vi "prepare_inserts_for_save_results.vi"(6 "operation_ID":string, 7 "SQL_connection_reference":T1, 8 "error_in":errorcluster, 9 "station":T2, 10 "results_from_PLC":T3, 11 "archivisation_info":string[][](array[string])) -> (0 "error_out":errorcluster, 3 "INSERT_statements":string[](array[string]), 5 "All PART_NUMBERS exist?":bool)   [LabVIEW 2020]
uses:
  ST_results_info.ctl
  station.ctl
  <vilib>/addons/database/Connection.llb/Conn ObjectReference.ctl
  FGV/SQL_batch_ID_buffer/FGV_SQL_batch_ID_buffer.ctl
  _misc/AULocalize/SubVIs/Get Localized Phrase Compact Interface 0D.vi
  <vilib>/addons/database/NI_Database_API.lvlib
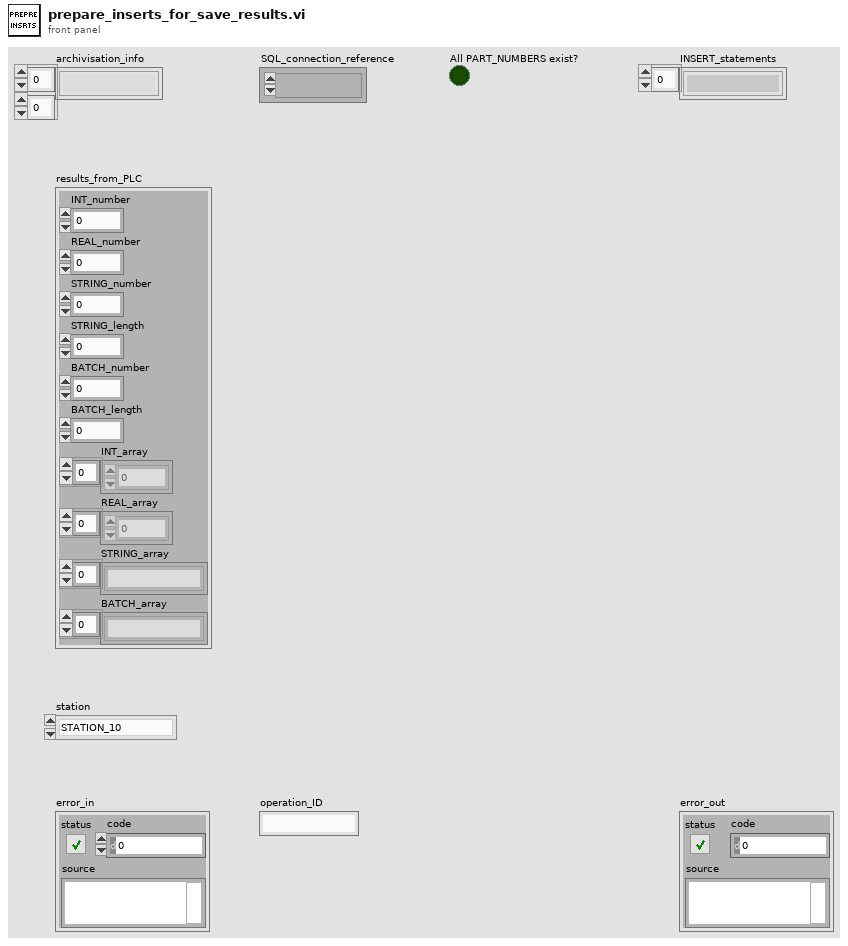
[diagram p1: front panel]
types:
  T1 = typedef "NI_Database_API.lvlib/Conn ObjectReference.ctl" = refnum<k1>
  T2 = typedef "station.ctl" = enum16{"STATION_10", "STATION_20", "STATION_30", "STATION_40", "STATION_50", "STATION_60", "STATION_70", "STATION_80", "STATION_90", "STATION_100", "STATION_110", "STATION_120", "STATION_165", "MAIN"}
  T3 = typedef "ST_results_info.ctl" = cluster{"INT_number":i32, "REAL_number":i32, "STRING_number":i32, "STRING_length":i32, "BATCH_number":i32, "BATCH_length":i32, "INT_array":i16[], "REAL_array":sgl[], "STRING_array":string[], "BATCH_array":string[]}
  T4 = typedef "FGV_SQL_batch_ID_buffer.ctl" = enum16{"initialize", "get_ID_for_number"}
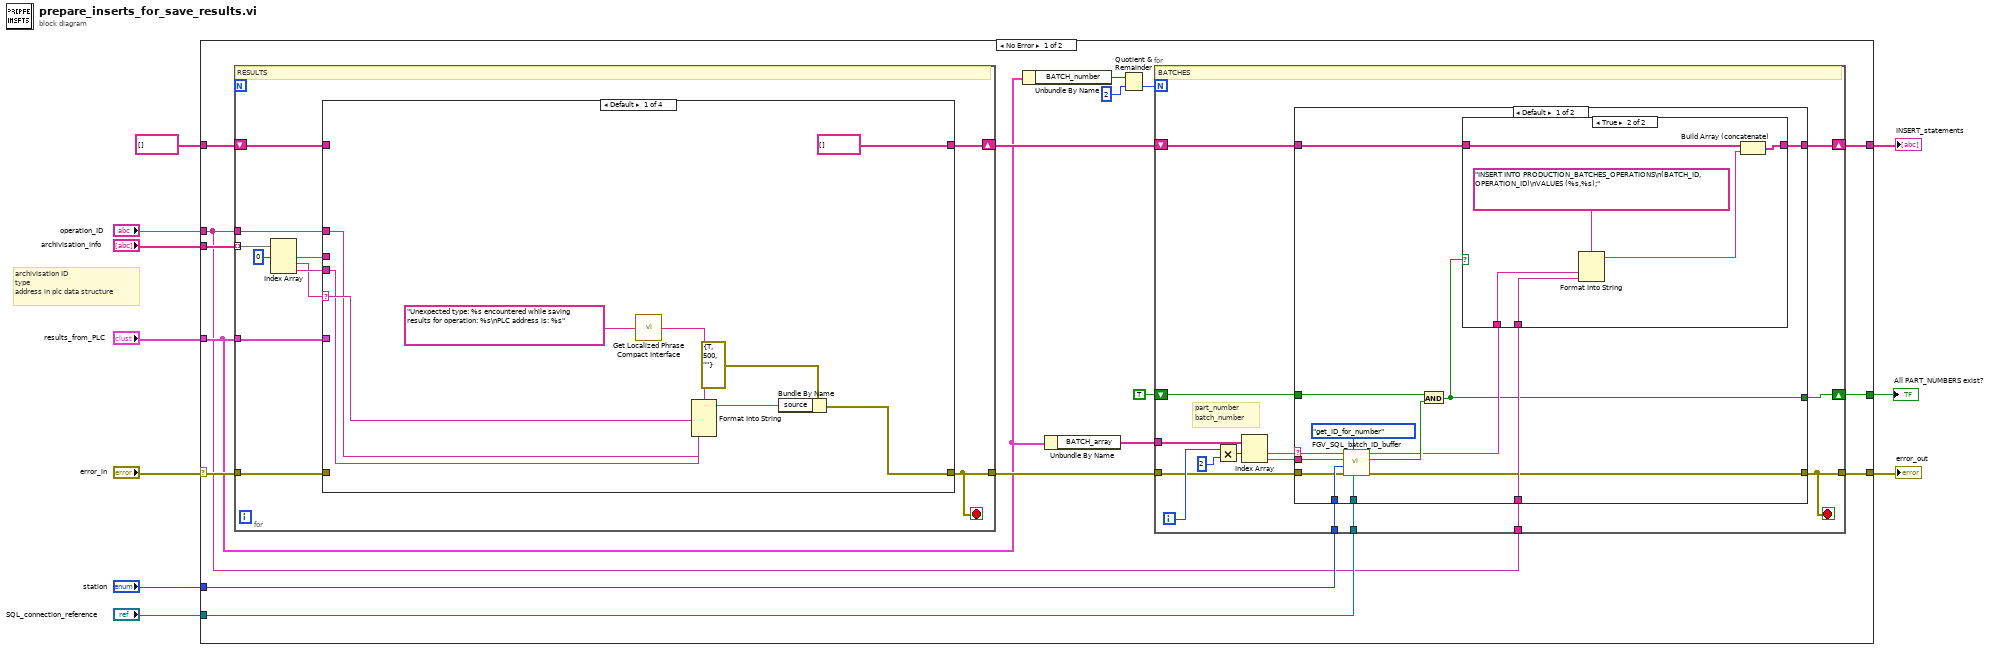
[diagram p0: block diagram]
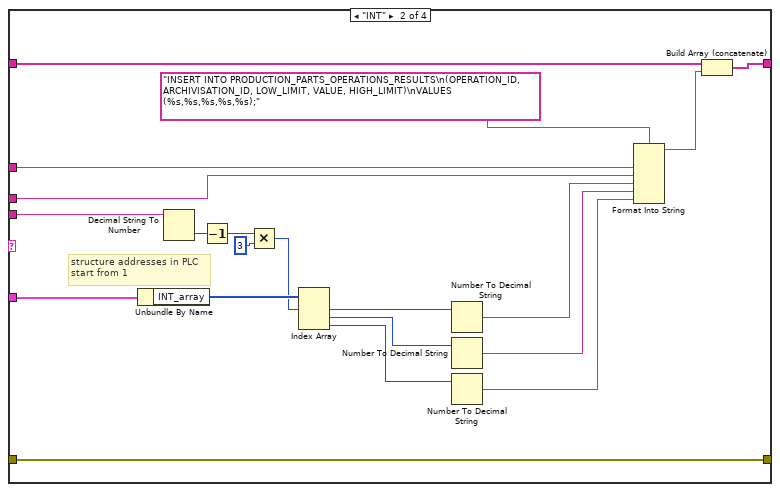
[diagram p4: hidden frame]
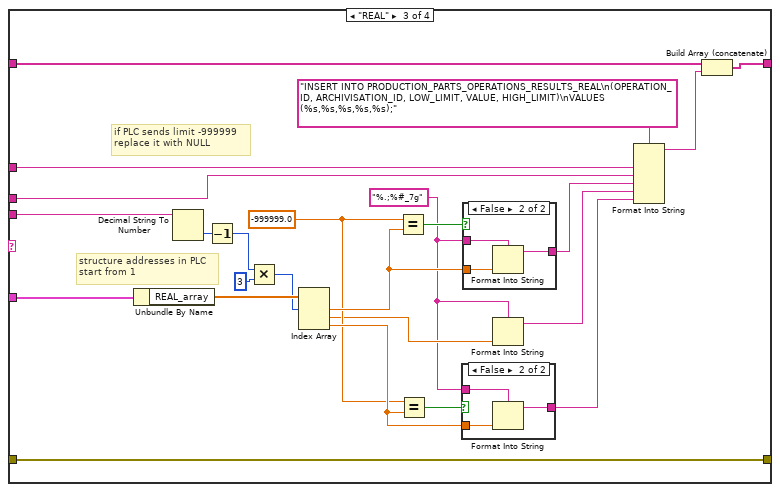
[diagram p5: hidden frame]
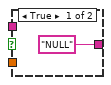
[diagram p6: hidden frame]
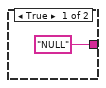
[diagram p7: hidden frame]
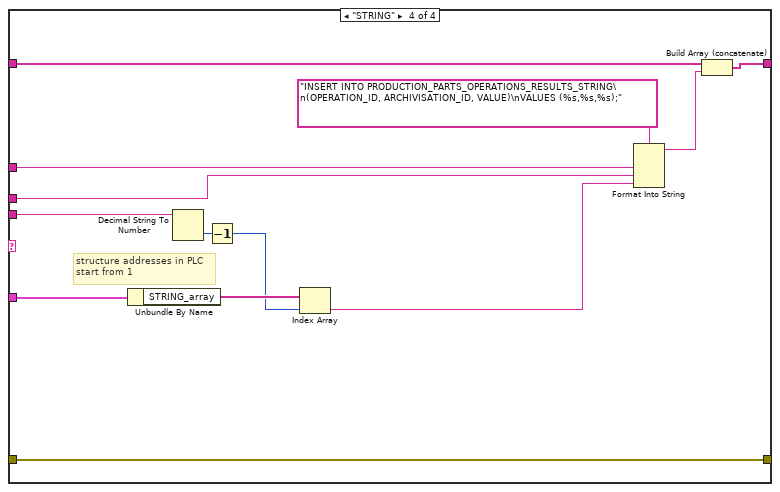
[diagram p8: hidden frame]
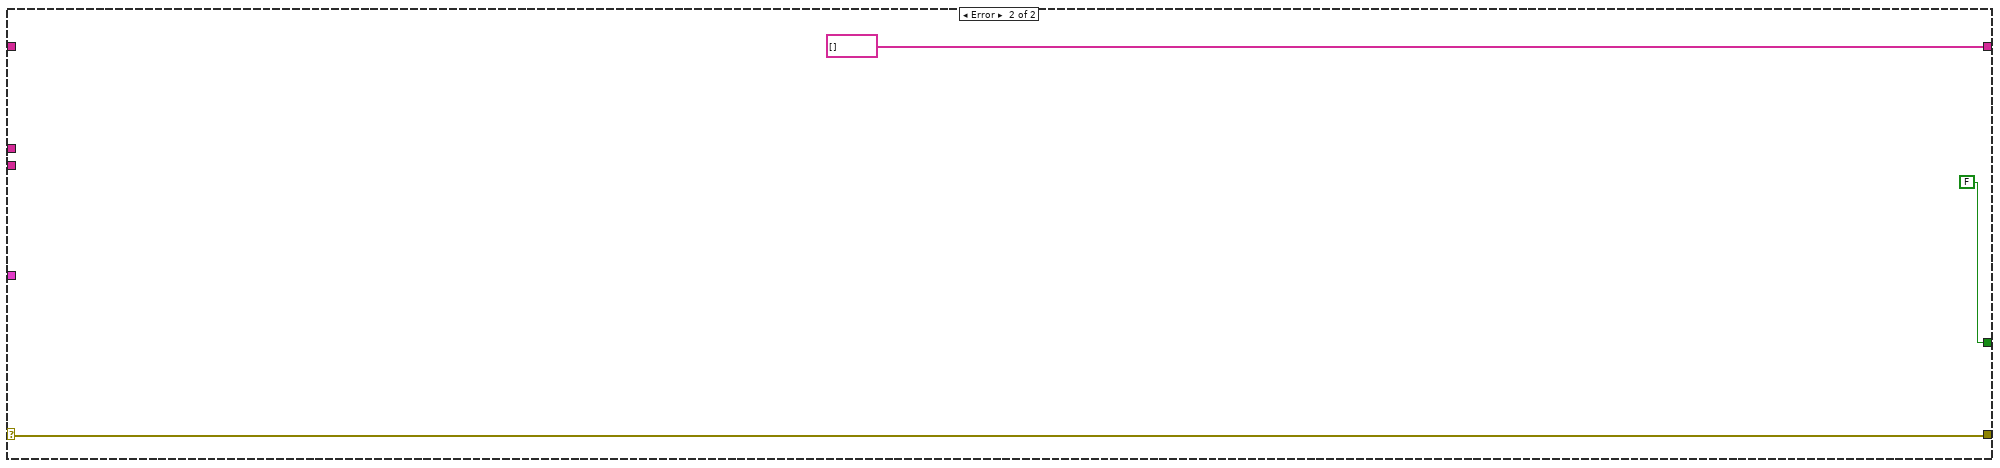
[diagram p9: hidden frame]
diagram:
  # "archivisation ID\ntype\naddress in plc data structure"
  n1 = case shown="No Error" "error_in" {
    selector: "error_in" -> [w25 w154]
    tunnel: "archivisation_info" -> [w27 _]
    tunnel: string[] [] ("INSERT_statements") -> [w26 _]
    tunnel: [w23 string[] [] ("INSERT_statements")] -> w8
    tunnel: "results_from_PLC" -> [w17 _]
    tunnel: "operation_ID" -> [w11 _]
    tunnel: [w21 w154] -> w4
    tunnel: "station" -> [w15 _]
    tunnel: "SQL_connection_reference" -> [w14 _]
    tunnel: [w12 FALSE] -> w1
    frame No Error {
      n2 = for {
        tunnel: w27 -> [w75] mode=indexing
        shift-right: [w76] -> w24
        shift-left: w26 -> [w77]
        tunnel: w17 -> [w71]
        tunnel: w11 -> [w72]
        tunnel: w25 -> [w68]
        tunnel: [w67] -> w22
        stop <- w67 stop-if-true
        # "RESULTS"
        n3 = Index Array(array=w75, index #1=0 ("index")) -> (element #1=w73:string, element #2=w69:string, element #3=w70:string)  [unwired: 2 in]
        n4 = case shown="Default" w69 {
          selector: w69 -> [w82 _ _ _]
          tunnel: w77 -> [_ w106 w130 w151]
          tunnel: [string[] [] w105 w129 w150] -> w76
          tunnel: w73 -> [_ w102 w126 w147]
          tunnel: w72 -> [w79 w101 w125 w146]
          tunnel: w71 -> [_ w100 w124 w145]
          tunnel: w70 -> [w80 w99 w123 w144]
          tunnel: w68 -> [_ w89 w118 w142]
          tunnel: [w84 w89 w118 w142] -> w67
          frame Default {
            n5 = call-poly "Get Localized Phrase Compact Interface.vi"("Key"="Unexpected type: %s encountered while saving results for operation: %s\nPLC address is: %s" ("source")) -> ("Translated Phrase"=w78:string)
            n6 = Format Into String(format string=w78, w82, w79, w80) -> (resulting string=w83:string)  [unwired: 2 in, 1 out]
            n7 = Bundle By Name(cluster=errorcluster {"status"=TRUE, "code"=500, "source"=""} ("error IO"), "source"=w83) -> (w84:errorcluster)
          }
          frame "INT" {
            # "structure addresses in PLC\nstart from 1"
            n8 = Unbundle By Name(w100) -> ("INT_array"=w95:i16[])
            n9 = Decimal String To Number(string=w99) -> (number=w88:i32)  [unwired: 2 in, 1 out]
            n10 = Decrement(x=w88) -> (x-1=w87:i32)
            n11 = Multiply(x=w87, y=3) -> (x*y=w93:i32)
            n12 = Index Array(array=w95, index #1=w93) -> (element #1=w92:i16, element #2=w91:i16, element #3=w90:i16)  [unwired: 2 in]
            n13 = Number To Decimal String(number=w92) -> (decimal integer string=w98:string)  [unwired: 1 in]
            n14 = Number To Decimal String(number=w91) -> (decimal integer string=w97:string)  [unwired: 1 in]
            n15 = Number To Decimal String(number=w90) -> (decimal integer string=w96:string)  [unwired: 1 in]
            n16 = Format Into String(format string="INSERT INTO PRODUCTION_PARTS_OPERATIONS_RESULTS\n(OPERATION_ID, ARCHIVISATION_ID, LOW_LIMIT, VALUE, HIGH_LIMIT)\nVALUES (%s,%s,%s,%s,%s);", w101, w102, w98, w97, w96) -> (resulting string=w103:string)  [unwired: 2 in, 1 out]
            n17 = Build Array (concatenate)(w106, w103) -> (w105:string[])
          }
          frame "REAL" {
            w107 = "%.;%#_7g" ("format string")
            w112 = sgl -999999.0 ("x")
            # "structure addresses in PLC\nstart from 1"
            # "if PLC sends limit -999999\nreplace it with NULL"
            n18 = Unbundle By Name(w124) -> ("REAL_array"=w121:sgl[])
            n19 = Decimal String To Number(string=w123) -> (number=w111:i32)  [unwired: 2 in, 1 out]
            n20 = Decrement(x=w111) -> (x-1=w110:i32)
            n21 = Multiply(x=w110, y=3) -> (x*y=w119:i32)
            n22 = Index Array(array=w121, index #1=w119) -> (element #1=w116:sgl, element #2=w108:sgl, element #3=w113:sgl)  [unwired: 2 in]
            n23 = Equal?(x=w112, y=w116) -> (x = y?=w117:bool)
            n24 = Equal?(x=w112, y=w113) -> (x = y?=w114:bool)
            n25 = case shown="False" w114 {
              tunnel: ["NULL" w134] -> w115
              tunnel: w113 -> [_ w133]
              tunnel: w107 -> [_ w132]
              frame True {
              }
              frame False {
                n26 = Format Into String(format string=w132, w133) -> (resulting string=w134:string)  [unwired: 2 in, 1 out]
              }
            }
            n27 = case shown="False" w117 {
              tunnel: ["NULL" w137] -> w122
              tunnel: w116 -> [_ w138]
              tunnel: w107 -> [_ w136]
              frame True {
              }
              frame False {
                n28 = Format Into String(format string=w136, w138) -> (resulting string=w137:string)  [unwired: 2 in, 1 out]
              }
            }
            n29 = Format Into String(format string=w107, w108) -> (resulting string=w109:string)  [unwired: 2 in, 1 out]
            n30 = Format Into String(format string="INSERT INTO PRODUCTION_PARTS_OPERATIONS_RESULTS_REAL\n(OPERATION_ID, ARCHIVISATION_ID, LOW_LIMIT, VALUE, HIGH_LIMIT)\nVALUES (%s,%s,%s,%s,%s);", w125, w126, w122, w109, w115) -> (resulting string=w127:string)  [unwired: 2 in, 1 out]
            n31 = Build Array (concatenate)(w130, w127) -> (w129:string[])
          }
          frame "STRING" {
            # "structure addresses in PLC\nstart from 1"
            n32 = Unbundle By Name(w145) -> ("STRING_array"=w143:string[])
            n33 = Decimal String To Number(string=w144) -> (number=w141:i32)  [unwired: 2 in, 1 out]
            n34 = Decrement(x=w141) -> (x-1=w140:i32)
            n35 = Index Array(array=w143, index=w140) -> (element=w139:string)
            n36 = Format Into String(format string="INSERT INTO PRODUCTION_PARTS_OPERATIONS_RESULTS_STRING\n(OPERATION_ID, ARCHIVISATION_ID, VALUE)\nVALUES (%s,%s,%s);", w146, w147, w139) -> (resulting string=w148:string)  [unwired: 2 in, 1 out]
            n37 = Build Array (concatenate)(w151, w148) -> (w150:string[])
          }
        }
      }
      n38 = Unbundle By Name(w17) -> ("BATCH_number"=w20:i32)
      n39 = Unbundle By Name(w17) -> ("BATCH_array"=w16:string[])
      n40 = Quotient & Remainder(x=w20, y=2) -> (floor(x/y)=w18:i32)  [unwired: 1 out]
      n41 = for {
        N: w18 -> [_]
        shift-right: [w36] -> w23
        shift-left: w24 -> [w37]
        tunnel: w22 -> [w29]
        tunnel: [w28] -> w21
        tunnel: w16 -> [w42]
        tunnel: w15 -> [w34]
        tunnel: w14 -> [w33]
        shift-right: [w32] -> w12
        shift-left: TRUE -> [w31]
        tunnel: w11 -> [w30]
        i -> [w40]
        stop <- w28 stop-if-true
        # "part_number\nbatch_number"
        # "BATCHES"
        n42 = Multiply(x=w40, y=2) -> (x*y=w41:i32)
        n43 = Index Array(array=w42, index #1=w41) -> (element #1=w38:string, element #2=w35:string)  [unwired: 1 in]
        n44 = case shown="Default" w38 {
          selector: w38 -> [w55 _]
          tunnel: w37 -> [w49 w66]
          tunnel: [w48 w66] -> w36
          tunnel: w35 -> [w54 _]
          tunnel: w34 -> [w56 _]
          tunnel: w33 -> [w52 _]
          tunnel: [w45 w65] -> w32
          tunnel: w31 -> [w50 w65]
          tunnel: w30 -> [w47 _]
          tunnel: w29 -> [w44 w64]
          tunnel: [w43 w64] -> w28
          frame Default {
            n45 = call "FGV_SQL_batch_ID_buffer.vi"("connection reference"=w52, "options"=FGV_SQL_batch_ID_buffer."get_ID_for_number", "error_in"=w44, "station"=w56, "BATCH_NUMBER"=w54, "PART_NUMBER"=w55) -> ("error_out"=w43:errorcluster, "PART_NUMBER exists?"=w51:bool, "ID_out"=w46:string)  [unwired: 3 in]
            n46 = And(x=w50, y=w51) -> (x .and. y?=w45:bool)
            n47 = case shown="True" w45 {
              tunnel: w49 -> [w57 w63]
              tunnel: [w57 w62] -> w48
              tunnel: w47 -> [_ w59]
              tunnel: w46 -> [_ w58]
              frame False {
              }
              frame True {
                n48 = Format Into String(format string="INSERT INTO PRODUCTION_BATCHES_OPERATIONS\n(BATCH_ID, OPERATION_ID)\nVALUES (%s,%s);", w58, w59) -> (resulting string=w60:string)  [unwired: 2 in, 1 out]
                n49 = Build Array (concatenate)(w63, w60) -> (w62:string[])
              }
            }
          }
          frame "" {
          }
        }
      }
    }
    frame Error {
    }
  }
  "INSERT_statements" <- w8
  "error_out" <- w4
  "All PART_NUMBERS exist?" <- w1
